vi "Get Tx Generic Frame Channels.vi"(8 "error in":errorcluster, 11 "Tx generic ref":T1 format="%.0x") -> (0 "error out":errorcluster, 2 "Tx generic frame channels":T1[](array[typedef]) format="%.0x", 3 "Tx generic ref out":T1 format="%.0x", 4 "found?":bool)   [LabVIEW 2020, in "AIM ARINC 664 Scripting.lvlib"]
uses:
  AIM ARINC 664 Scripting.lvlib
  Constants.vi
  <vilib>/NI VeriStand/Custom Device Tools/Custom Device Utility Library/Custom Device Utility Library.lvlib
  <vilib>/NI VeriStand/Custom Device Tools/Custom Device Utility Library/NI VeriStand - Search for All Items by GUID.vi
  <vilib>/NI VeriStand/Custom Device API/Custom Device Item Ref.ctl
  <vilib>/NI VeriStand/Custom Device API/Custom Device API.lvlib
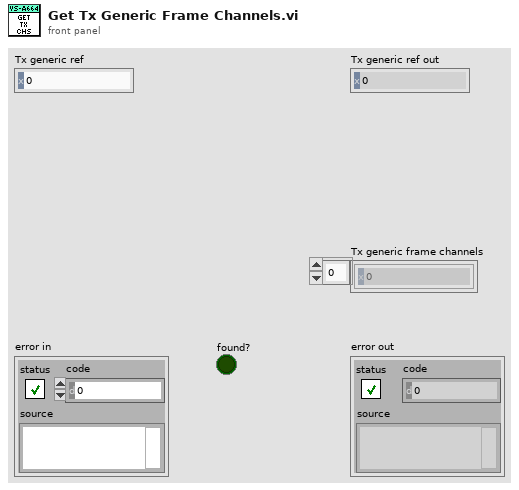
[diagram p1: front panel]
types:
  T1 = typedef "Custom Device API.lvlib/Custom Device Item Ref.ctl" = u64
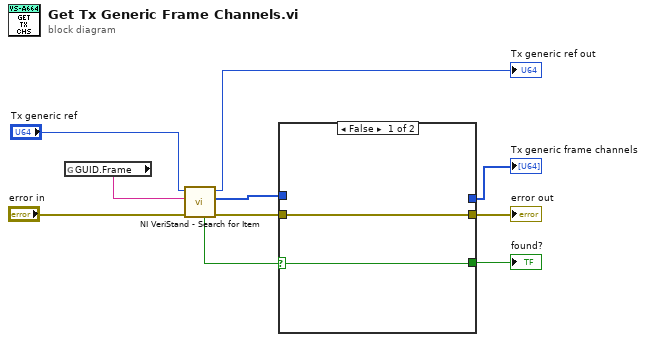
[diagram p0: block diagram]
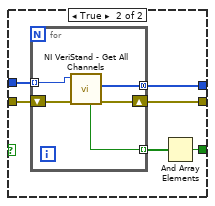
[diagram p2: hidden frame]
diagram:
  n1 = global read "Constants.vi" "GUID.Frame"() -> (w9:string)
  n2 = call-poly <vilib>:"NI VeriStand - Search for Item.vi"("error in"="error in", "Item GUID"=w9, "Section Ref in"="Tx generic ref") -> ("error out"=w6:errorcluster, "Item Refs"=w4:T1[], "Section Ref out"=→"Tx generic ref out":T1, "Found"=w5:bool)  [unwired: 5 in]
  n3 = case shown="False" w5 {
    selector: w5 -> [w11 _]
    tunnel: w6 -> [w12 w18]
    tunnel: w4 -> [_ w17]
    tunnel: [_ w16] -> w2
    tunnel: [w12 w15] -> w3
    tunnel: [w11 w13] -> w1
    frame False {
    }
    frame True {
      n4 = for {
        shift-right: [w21] -> w15
        shift-left: w18 -> [w23]
        tunnel: w17 -> [w22] mode=indexing
        tunnel: [w20] -> w16 mode=concatenating
        tunnel: [w19] -> w14 mode=indexing
        n5 = call <vilib>:"NI VeriStand - Get All Channels.vi"("error in"=w23, "Section Ref in"=w22) -> ("error out"=w21:errorcluster, "Channel Refs"=w20:T1[], "Found"=w19:bool)  [unwired: 6 in, 1 out]
      }
      n6 = And Array Elements(Boolean array=w14) -> (logical AND=w13:bool)
    }
  }
  "error out" <- w3
  "Tx generic frame channels" <- w2
  "found?" <- w1
